vi "Get JSON API Documentation.vi"(8 "error in (no error)":errorcluster, 10 "Help cluster":T1, 11 "Help":refnum<class "Help.lvclass">) -> (0 "error out":errorcluster, 2 "<JSON> API doc":string, 3 "Help out":refnum<class "Help.lvclass">)   [LabVIEW 2019, in "Instrument.lvlib" / "Help.lvclass"]
uses:
  Help.lvclass
  typedefs/Help--cluster.ctl
  Help.lvclass/Help.ctl
  <vilib>/JDP Science/JSONtext/JSONtext.lvlib
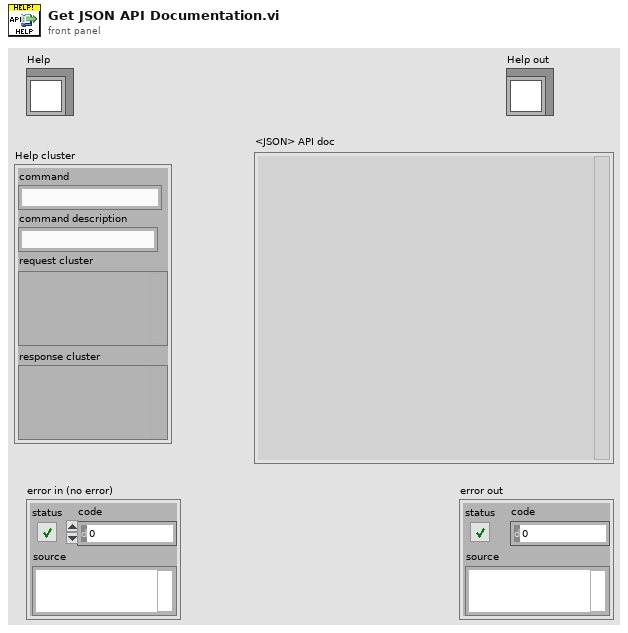
[diagram p1: front panel]
types:
  T1 = typedef "Instrument.lvlib/Help.lvclass/Help--cluster.ctl" = cluster{"command":string, "command description":string, "request cluster":variant, "response cluster":variant}
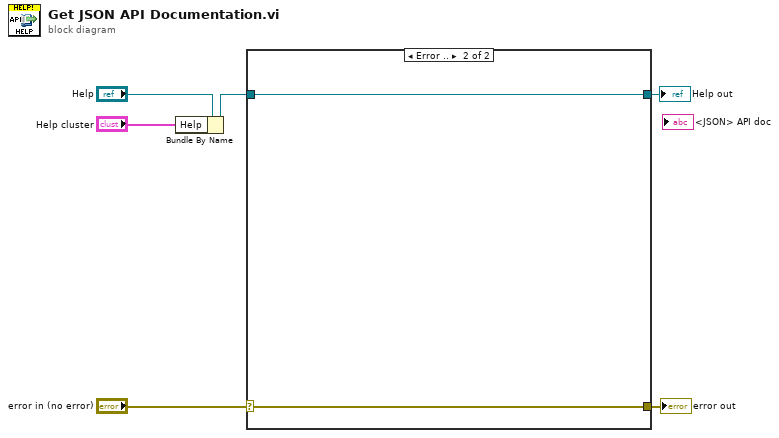
[diagram p0: block diagram]
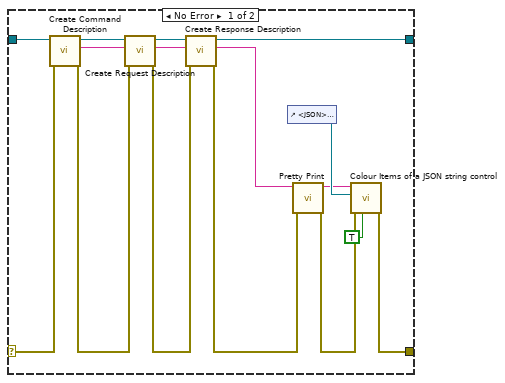
[diagram p2: hidden frame]
diagram:
  n1 = Bundle By Name(cluster="Help", "Help"="Help cluster") -> (w2:refnum<class "Help.lvclass">)
  n2 = case shown="Error .." "error in (no error)" {
    selector: "error in (no error)" -> [w15 w24]
    tunnel: [w17 w24] -> w5
    tunnel: w2 -> [w11 w23]
    tunnel: [w8 w23] -> w4
    frame No Error {
      n3 = call "Create Command Description.vi"("error in (no error)"=w15, "Help in"=w11) -> ("error out"=w18:errorcluster, "<JSON> out"=w19:string, "Help out"=w10:refnum<class "Help.lvclass">)  [unwired: 7 in]
      n4 = call "Create Request Description.vi"("error in (no error)"=w18, "JSON in"=w19, "Help in"=w10) -> ("error out"=w12:errorcluster, "<JSON> out"=w13:string, "Help out"=w9:refnum<class "Help.lvclass">)  [unwired: 6 in]
      n5 = call "Create Response Description.vi"("error in (no error)"=w12, "JSON in"=w13, "Help in"=w9) -> ("error out"=w14:errorcluster, "<JSON> out"=w7:string, "Help out"=w8:refnum<class "Help.lvclass">)  [unwired: 6 in]
      n6 = control-ref of="<JSON> API doc"() -> (w22:refnum<vi>)
      n7 = call <vilib>:"Pretty Print.vi"("error in (no error)"=w14, "JSON"=w7) -> ("error out"=w20:errorcluster, "<JSON>"=w16:string)  [unwired: 7 in, 1 out]
      n8 = call <vilib>:"Colour Items of a JSON string control.vi"("Defer Panel Updates"=TRUE, "error in (no error)"=w20, "String Control"=w22, "JSON"=w16) -> ("error out"=w17:errorcluster)  [unwired: 7 in]
    }
    frame Error {
    }
  }
  "error out" <- w5
  "Help out" <- w4
